vi "PQfetchResultData.vi"(8 "error in":errorcluster, 10 "res":u32, 11 "conn":u32) -> (0 "error out":errorcluster, 1 "Data":string[][](array[string]), 2 "res_out":u32, 3 "conn_out":u32, 4 "PQnFields":i32, 6 "PQnTuples":i32)   [LabVIEW 2019, in "libpqutility.lvlib"]
doc: "Fetch Result Data from DatabaseRequest into String Array.\nSee PostgreSQL c-lib doku for further information."
uses:
  libpqutility.lvlib
  libpqlv/libpqlv.lvlib
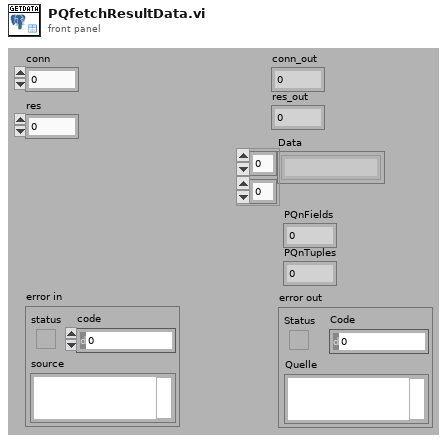
[diagram p1: front panel]
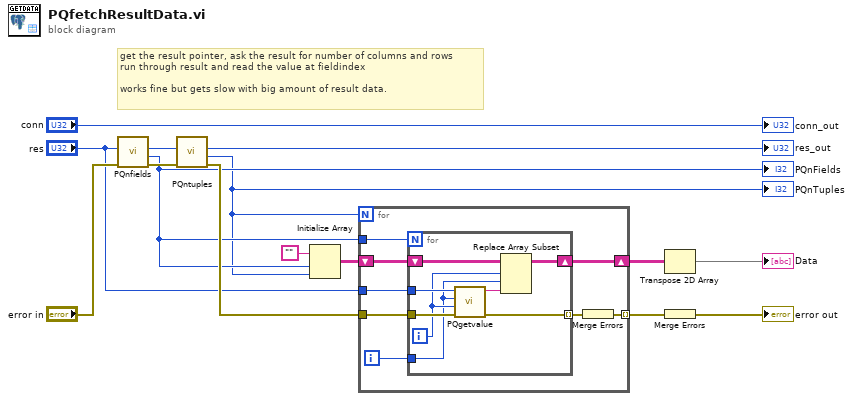
[diagram p0: block diagram]
diagram:
  # "get the result pointer, ask the result for number of columns and rows\nrun through result and read the value at fieldindex\n\nworks fine but gets slow with big amount of result data."
  n1 = call "PQnfields.vi"("error in (no error)"="error in", "res"="res") -> ("error out"=w13:errorcluster, "PQnFields"=w6:i32, "res out"=w2:u32)  [unwired: 7 in]
  "PQnFields" <- w6
  n2 = call "PQntuples.vi"("error in (no error)"=w13, "res"=w2) -> ("error out"=w12:errorcluster, "PQnTuples"=w5:i32, "res out"=→"res_out":u32)  [unwired: 7 in]
  "PQnTuples" <- w5
  n3 = Initialize Array("", w6, w5) -> (w7:string[][])
  n4 = for {
    N: w5 -> [_]
    tunnel: "res" -> [w23]
    tunnel: w6 -> [w20]
    tunnel: w12 -> [w21]
    tunnel: [w16] -> w4 mode=indexing
    shift-right: [w19] -> w9
    shift-left: w7 -> [w18]
    i -> [w22]
    n5 = for {
      N: w20 -> [_]
      tunnel: w23 -> [w31]
      tunnel: w22 -> [w27]
      tunnel: w21 -> [w30]
      tunnel: [w29] -> w17 mode=indexing
      shift-right: [w25] -> w19
      shift-left: w18 -> [w24]
      i -> [w28]
      n6 = call "PQgetvalue.vi"("error in (no error)"=w30, "column_number"=w28, "row_number"=w27, "res"=w31) -> ("error out"=w29:errorcluster, "field_value"=w26:string)  [unwired: 6 in]
      n7 = Replace Array Subset(array=w24, new element=w26, index (row)=w28, index (col)=w27) -> (w25:string[][])
    }
    n8 = Merge Errors(w17) -> (w16:errorcluster)
  }
  n9 = Transpose 2D Array(2D array=w9) -> (transposed array=→"Data":string[][])
  n10 = Merge Errors(w4) -> (→"error out":errorcluster)
  "conn_out" <- "conn"
